vi "TextToVariant.vi"(7 "Data Type":variant, 8 "error in (no error)":errorcluster, 10 "Serializable Text":string, 11 "BlueJSONTextSerializer in":refnum<class "BlueJSONTextSerializer.lvclass">) -> (0 "error out":errorcluster, 2 "Variant out":variant, 3 "BlueJSONTextSerializer out":refnum<class "BlueJSONTextSerializer.lvclass">)   [LabVIEW 2019, in "BlueJSONTextSerializer.lvlib" / "BlueJSONTextSerializer.lvclass"]
uses:
  BlueJSONTextSerializer.lvclass
  <vilib>/JDP Science/JSONtext/JSONtext.lvlib
  BlueJSONtext LVClass Serializer/BlueJSONtext LVClass Serializer.lvclass
  C:/Program Files (x86)/National Instruments/LabVIEW 2019/vi.lib/JDP Science/JSONtext/LVClass Serializer/JSONtext LVClass Serializer.lvclass
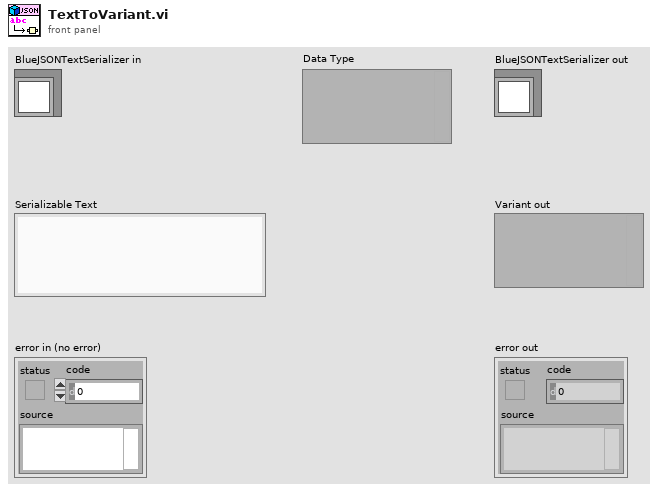
[diagram p1: front panel]
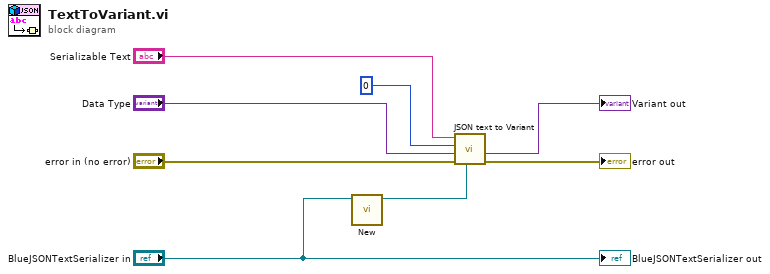
[diagram p0: block diagram]
diagram:
  n1 = call "New.vi"("BlueJSONTextSerializer"="BlueJSONTextSerializer in") -> ("BlueJSONtext LVClass Serializer out"=w1:refnum<class "BlueJSONtext LVClass Serializer.lvclass">)  [unwired: 10 in]
  n2 = call <vilib>:"JSON text to Variant.vi"("LVClass Serializer"=w1, "error in (no error)"="error in (no error)", "Data Type"="Data Type", "Offset"=0, "JSON"="Serializable Text") -> ("error out"=→"error out":errorcluster, "Variant out"=→"Variant out":variant)  [unwired: 5 in]
  "BlueJSONTextSerializer out" <- "BlueJSONTextSerializer in"
